vi "Open Data Logging Manager Reference.vi"(8 "error in (no error)":errorcluster, 11 "Gateway IP Address (\"\": localhost)":string) -> (0 "error out":errorcluster, 3 "Data Logging Manager Ref out":T1)   [LabVIEW 2020, in "NI_VS Data Logging API.lvlib"]
doc: "Opens a connection to the data logging service on the VeriStand Gateway. You must open a reference to the Data Logging Manager to enable the host computer to log data from a target while a system definition is deployed and running."
uses:
  <vilib>/NI VeriStand/Execution/DataLogging/NI_VS Data Logging API.lvlib
  <vilib>/NI VeriStand/Execution/DataLogging/IDataLogging Ref.ctl
  NationalInstruments.VeriStand.ClientAPI
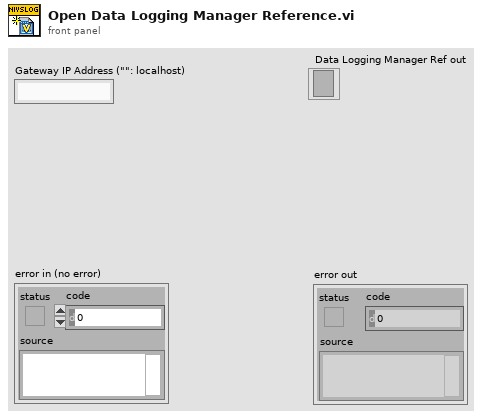
[diagram p1: front panel]
types:
  T1 = typedef "NI_VS Data Logging API.lvlib/IDataLogging Ref.ctl" = refnum<k24>
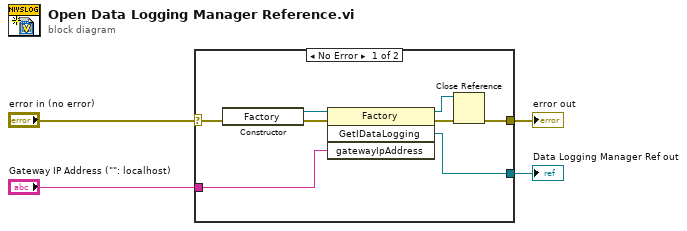
[diagram p0: block diagram]
diagram:
  n1 = case shown="No Error" "error in (no error)" {
    selector: "error in (no error)" -> [w12 w13]
    tunnel: "Gateway IP Address (\"\": localhost)" -> [w9 _]
    tunnel: [w6 w13] -> w2
    tunnel: [w5 _] -> w1
    frame No Error {
      n2 = constructor class="Factory"(error in=w12) -> (reference out=w10:refnum<k24>, error out=w11:errorcluster)  [unwired: 2 in, 1 out]
      n3 = invoke class="Factory" method="GetIDataLogging"(reference=w10, error in=w11, "gatewayIpAddress"=w9) -> (reference out=w7:refnum<k24>, error out=w8:errorcluster, "GetIDataLogging"=w5:refnum<k24>)  [unwired: 1 in, 1 out]
      n4 = Close Reference(reference=w7, error in (no error)=w8) -> (error out=w6:errorcluster)
    }
    frame Error {
    }
  }
  "Data Logging Manager Ref out" <- w1
  "error out" <- w2
